vi "Use Application Directory if Input is Empty.vi"(1 "Directory(Use Application Directory if Input is Empty)":path) -> (0 "Directory":path)   [LabVIEW 2017]
doc: "Returns Directory unchanged, and substitutes the application directory when the input path is empty."
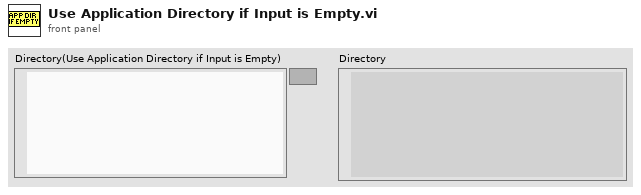
[diagram p1: front panel]
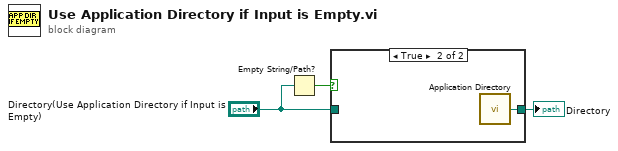
[diagram p0: block diagram]
diagram:
  n1 = Empty String/Path?(string/path="Directory(Use Application Directory if Input is Empty)") -> (empty?=w1:bool)
  n2 = case shown="True" w1 {
    tunnel: [w4 w5] -> w2
    tunnel: "Directory(Use Application Directory if Input is Empty)" -> [w4 _]
    frame False {
    }
    frame True {
      n3 = call <vilib>:"Application Directory.vi"() -> ("Application Directory"=w5:path)
    }
  }
  "Directory" <- w2
